vi "CalcArmCurlSpeed.vi"(9 "Curl Speed":dbl, 10 "Elbow Down":bool, 11 "Elbow Up":bool) -> (2 "Elbow Speed":dbl, 3 "Shoulder Speed":dbl)   [LabVIEW 2018]
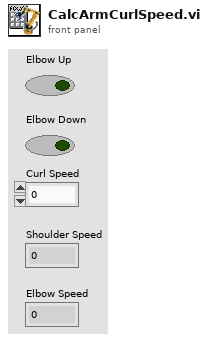
[diagram p1: front panel]
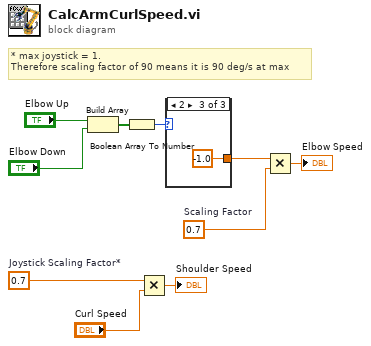
[diagram p0: block diagram]
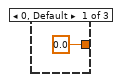
[diagram p2: hidden frame]
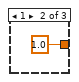
[diagram p3: hidden frame]
diagram:
  w3 = 0.7  # Scaling Factor
  w10 = 0.7  # Joystick Scaling Factor*
  # "* max joystick = 1.\nTherefore scaling factor of 90 means it is 90 deg/s at max"
  n1 = Build Array("Elbow Up", "Elbow Down") -> (w7:bool[])
  n2 = Boolean Array To Number(Boolean array=w7) -> (number=w4:u32)
  n3 = Multiply(x=w10, y="Curl Speed") -> (x*y=→"Shoulder Speed":dbl)
  n4 = case shown="2" w4 {
    tunnel: [0.0 1.0 -1.0] -> w2
    frame 0, Default {
    }
    frame 1 {
    }
    frame 2 {
    }
  }
  n5 = Multiply(x=w2, y=w3) -> (x*y=→"Elbow Speed":dbl)
